vi "test-diff-drive-kinematics.vi"() -> ()   [LabVIEW 2019]
uses:
  <vilib>/Rock Robotics/SystemInterfaces/NetworkCommunication/NetComm_UsageReport_report.vi
  <vilib>/Rock Robotics/WPI/ThirdParty/JAS_Junk/TrajLib/Util_LibraryGlobals.vi
  <vilib>/Rock Robotics/WPI/ThirdParty/JAS_Junk/TrajLib/Trajectory_Library.lvlib
panel:
  out "T5 -- Omega = 0":dbl
  out "T5 -- Y = 0":dbl
  out "T5 -- X = 0":dbl
  out "T4 -- Right = 0":dbl
  out "T4 -- Left = 0":dbl
  out "T3 -- Omega = 0":dbl
  out "T3 -- Y = 0":dbl
  out "T3 -- X = 0":dbl
  out "T2 -- Right = 0":dbl
  out "T2 -- Left = 0":dbl
  out "T1 -- Omega = 0":dbl
  out "T0 -- Y = 0":dbl
  out "T0 -- X = 0":dbl
  out "T1 -- Right = 0":dbl
  out "T1 -- Left = 0":dbl
  # "Diff Drive Kinematic Test"
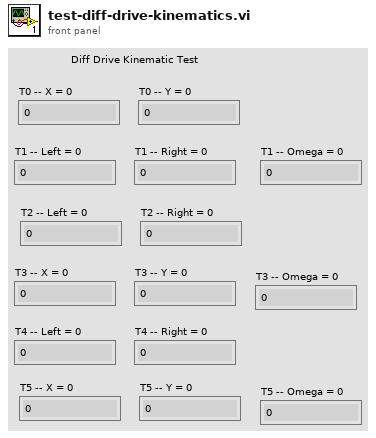
[diagram p1: front panel]
types:
  T1 = typedef "Trajectory_Library.lvlib/CHASSIS_SPEEDS.ctl" = cluster{"vX":dbl, "vY":dbl, "vOmega":dbl}
  T2 = typedef "Trajectory_Library.lvlib/DIFF_DRIVE_KINEMATICS.ctl" = cluster{"TrackWidth_Meters":dbl}
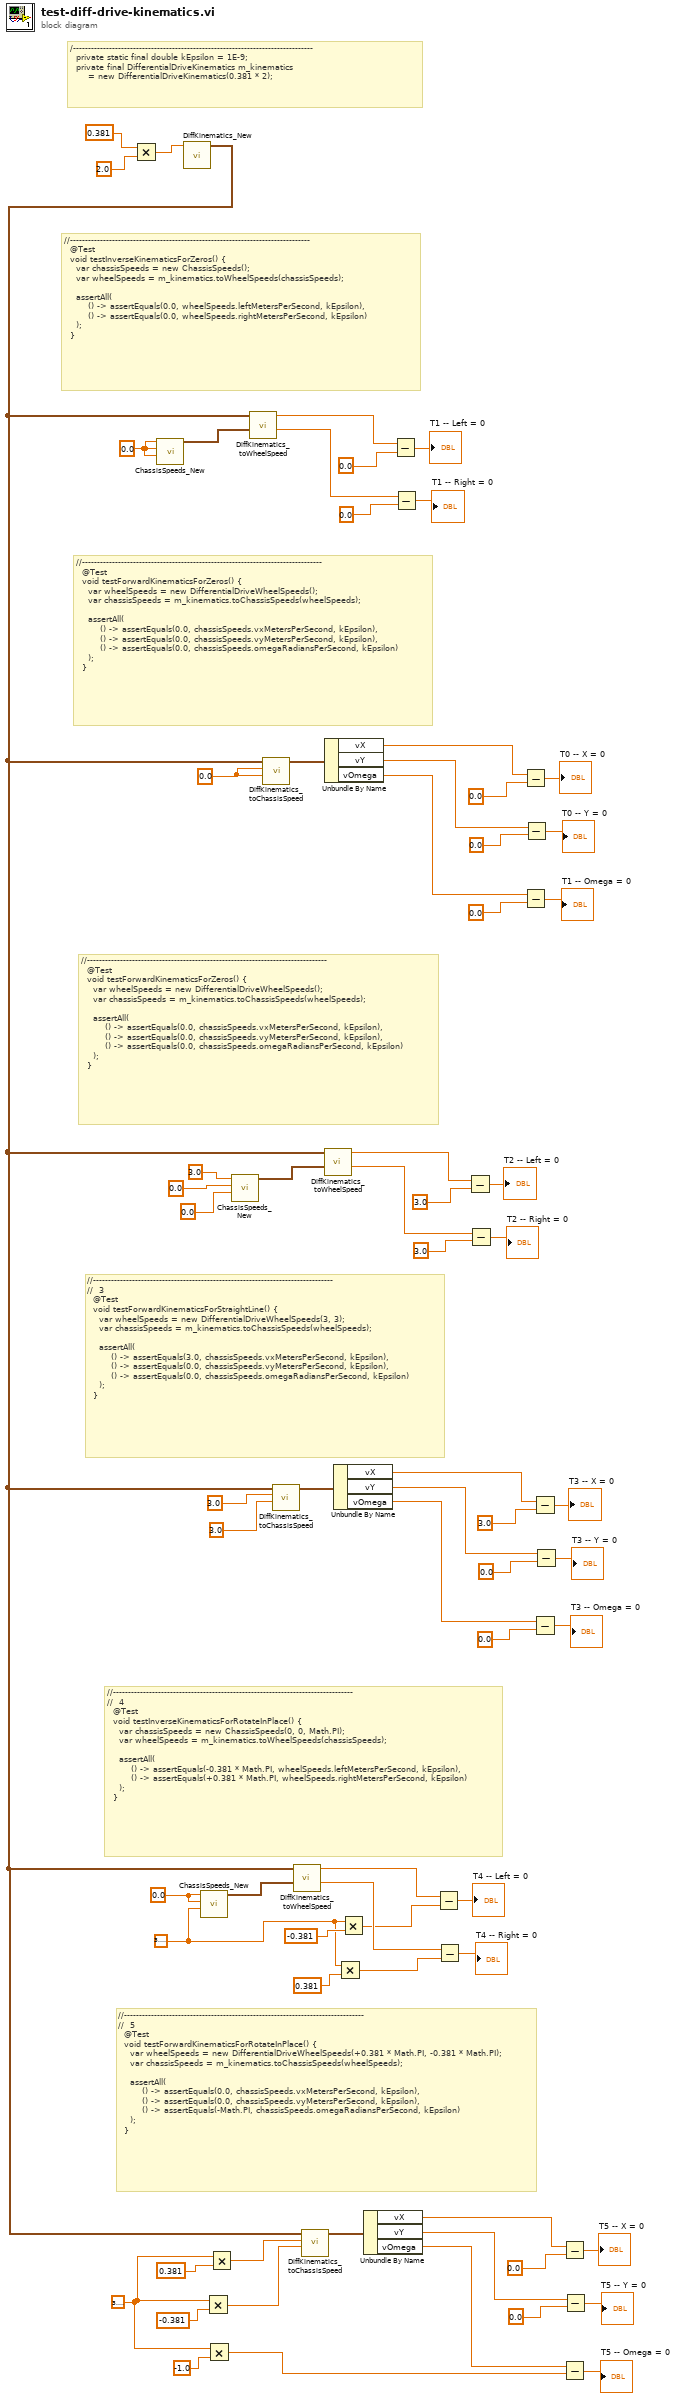
[diagram p0: block diagram]
diagram:
  w2 = 3.141592653589793
  w20 = 3.141592653589793
  w26 = 0.0 ("vX")
  w61 = 0.0 ("LeftVelocity")
  w65 = 0.0 ("vX")
  # "//--------------------------------------------------------------------------------\n//  5\n  @Test\n  void testForwardKinematicsForRotateInPlace() {\n    var wheelSpeeds = new DifferentialDriveWheelSpeeds(+0.381 * Math.PI, -0.381 * Math.PI);\n    var chassisSpeeds = m_kinematics.toChassisSpeeds(wheelSpeeds);\n\n    assertAll(\n        () -> assertEquals(0.0, chassisSpeeds.vxMetersPerSecond, kEpsilon),\n        () -> assertEquals(0.0, chassisSpeeds.vyMetersPerSecond, kEpsilon),\n        () -> assertEquals(-Math.PI, chassisSpeeds.omegaRadiansPerSecond, kEpsilon)\n    );\n  }"
  # "//--------------------------------------------------------------------------------\n//  4\n  @Test\n  void testInverseKinematicsForRotateInPlace() {\n    var chassisSpeeds = new ChassisSpeeds(0, 0, Math.PI);\n    var wheelSpeeds = m_kinematics.toWheelSpeeds(chassisSpeeds);\n\n    assertAll(\n        () -> assertEquals(-0.381 * Math.PI, wheelSpeeds.leftMetersPerSecond, kEpsilon),\n        () -> assertEquals(+0.381 * Math.PI, wheelSpeeds.rightMetersPerSecond, kEpsilon)\n    );\n  }"
  # "//--------------------------------------------------------------------------------\n//  3\n  @Test\n  void testForwardKinematicsForStraightLine() {\n    var wheelSpeeds = new DifferentialDriveWheelSpeeds(3, 3);\n    var chassisSpeeds = m_kinematics.toChassisSpeeds(wheelSpeeds);\n\n    assertAll(\n        () -> assertEquals(3.0, chassisSpeeds.vxMetersPerSecond, kEpsilon),\n        () -> assertEquals(0.0, chassisSpeeds.vyMetersPerSecond, kEpsilon),\n        () -> assertEquals(0.0, chassisSpeeds.omegaRadiansPerSecond, kEpsilon)\n    );\n  }"
  # "//--------------------------------------------------------------------------------\n  @Test\n  void testForwardKinematicsForZeros() {\n    var wheelSpeeds = new DifferentialDriveWheelSpeeds();\n    var chassisSpeeds = m_kinematics.toChassisSpeeds(wheelSpeeds);\n\n    assertAll(\n        () -> assertEquals(0.0, chassisSpeeds.vxMetersPerSecond, kEpsilon),\n        () -> assertEquals(0.0, chassisSpeeds.vyMetersPerSecond, kEpsilon),\n        () -> assertEquals(0.0, chassisSpeeds.omegaRadiansPerSecond, kEpsilon)\n    );\n  }"
  # "//--------------------------------------------------------------------------------\n  @Test\n  void testForwardKinematicsForZeros() {\n    var wheelSpeeds = new DifferentialDriveWheelSpeeds();\n    var chassisSpeeds = m_kinematics.toChassisSpeeds(wheelSpeeds);\n\n    assertAll(\n        () -> assertEquals(0.0, chassisSpeeds.vxMetersPerSecond, kEpsilon),\n        () -> assertEquals(0.0, chassisSpeeds.vyMetersPerSecond, kEpsilon),\n        () -> assertEquals(0.0, chassisSpeeds.omegaRadiansPerSecond, kEpsilon)\n    );\n  }"
  # "/--------------------------------------------------------------------------------\n  private static final double kEpsilon = 1E-9;\n  private final DifferentialDriveKinematics m_kinematics\n      = new DifferentialDriveKinematics(0.381 * 2);"
  # "//--------------------------------------------------------------------------------\n  @Test\n  void testInverseKinematicsForZeros() {\n    var chassisSpeeds = new ChassisSpeeds();\n    var wheelSpeeds = m_kinematics.toWheelSpeeds(chassisSpeeds);\n\n    assertAll(\n        () -> assertEquals(0.0, wheelSpeeds.leftMetersPerSecond, kEpsilon),\n        () -> assertEquals(0.0, wheelSpeeds.rightMetersPerSecond, kEpsilon)\n    );\n  }"
  n1 = Multiply(x=0.381, y=2.0) -> (x*y=w66:dbl)
  n2 = call <vilib>:"ChassisSpeeds_New.vi"("vAngular"=w65, "vY"=w65, "vX"=w65) -> ("CHASSIS"=w64:T1)  [unwired: 8 in]
  n3 = call <vilib>:"DiffKinematics_New.vi"("TrackWidth_Meters"=w66) -> ("DIFF_DRIVE_KINEMATICS"=w8:T2)  [unwired: 10 in]
  n4 = call <vilib>:"ChassisSpeeds_New.vi"("vAngular"=w20, "vY"=w26, "vX"=w26) -> ("CHASSIS"=w25:T1)  [unwired: 8 in]
  n5 = Multiply(x=w2, y=-0.381) -> (x*y=w4:dbl)
  n6 = Multiply(x=w2, y=-1.0) -> (x*y=w1:dbl)
  n7 = Multiply(x=w2, y=0.381) -> (x*y=w5:dbl)
  n8 = call <vilib>:"ChassisSpeeds_New.vi"("vAngular"=0.0, "vY"=0.0, "vX"=3.0) -> ("CHASSIS"=w46:T1)  [unwired: 8 in]
  n9 = call <vilib>:"DiffKinematics_toWheelSpeed.vi"("CHASSIS Speed"=w64, "DIFF_DRIVE_KINEMATICS"=w8) -> ("RightVelocity"=w62:dbl, "LeftVelocity"=w63:dbl)  [unwired: 8 in]
  n10 = call <vilib>:"DiffKinematics_toChassisSpeed.vi"("RightVelocity"=w61, "LeftVelocity"=w61, "inDIFF_DRIVE_KINEMATICS"=w8) -> ("CHASSIS Speed"=w60:T1)  [unwired: 8 in]
  n11 = call <vilib>:"DiffKinematics_toChassisSpeed.vi"("RightVelocity"=3.0, "LeftVelocity"=3.0, "inDIFF_DRIVE_KINEMATICS"=w8) -> ("CHASSIS Speed"=w39:T1)  [unwired: 8 in]
  n12 = call <vilib>:"DiffKinematics_toWheelSpeed.vi"("CHASSIS Speed"=w25, "DIFF_DRIVE_KINEMATICS"=w8) -> ("RightVelocity"=w23:dbl, "LeftVelocity"=w24:dbl)  [unwired: 8 in]
  n13 = call <vilib>:"DiffKinematics_toChassisSpeed.vi"("RightVelocity"=w4, "LeftVelocity"=w5, "inDIFF_DRIVE_KINEMATICS"=w8) -> ("CHASSIS Speed"=w17:T1)  [unwired: 8 in]
  n14 = Unbundle By Name(w60) -> ("vX"=w53:dbl, "vY"=w52:dbl, "vOmega"=w51:dbl)
  n15 = call <vilib>:"DiffKinematics_toWheelSpeed.vi"("CHASSIS Speed"=w46, "DIFF_DRIVE_KINEMATICS"=w8) -> ("RightVelocity"=w44:dbl, "LeftVelocity"=w45:dbl)  [unwired: 8 in]
  n16 = Unbundle By Name(w39) -> ("vX"=w32:dbl, "vY"=w31:dbl, "vOmega"=w30:dbl)
  n17 = Multiply(x=w20, y=0.381) -> (x*y=w18:dbl)
  n18 = Multiply(x=w20, y=-0.381) -> (x*y=w19:dbl)
  n19 = Unbundle By Name(w17) -> ("vX"=w11:dbl, "vY"=w10:dbl, "vOmega"=w9:dbl)
  n20 = Subtract(x=w63, y=0.0) -> (x-y=→"T1 -- Left = 0":dbl)
  n21 = Subtract(x=w62, y=0.0) -> (x-y=→"T1 -- Right = 0":dbl)
  n22 = Subtract(x=w24, y=w19) -> (x-y=→"T4 -- Left = 0":dbl)
  n23 = Subtract(x=w23, y=w18) -> (x-y=→"T4 -- Right = 0":dbl)
  n24 = Subtract(x=w45, y=3.0) -> (x-y=→"T2 -- Left = 0":dbl)
  n25 = Subtract(x=w44, y=3.0) -> (x-y=→"T2 -- Right = 0":dbl)
  n26 = Subtract(x=w53, y=0.0) -> (x-y=→"T0 -- X = 0":dbl)
  n27 = Subtract(x=w51, y=0.0) -> (x-y=→"T1 -- Omega = 0":dbl)
  n28 = Subtract(x=w52, y=0.0) -> (x-y=→"T0 -- Y = 0":dbl)
  n29 = Subtract(x=w32, y=3.0) -> (x-y=→"T3 -- X = 0":dbl)
  n30 = Subtract(x=w30, y=0.0) -> (x-y=→"T3 -- Omega = 0":dbl)
  n31 = Subtract(x=w31, y=0.0) -> (x-y=→"T3 -- Y = 0":dbl)
  n32 = Subtract(x=w11, y=0.0) -> (x-y=→"T5 -- X = 0":dbl)
  n33 = Subtract(x=w9, y=w1) -> (x-y=→"T5 -- Omega = 0":dbl)
  n34 = Subtract(x=w10, y=0.0) -> (x-y=→"T5 -- Y = 0":dbl)
